vi "Q8381 QRY REF LEVEL.vi"(0 "VISA resource name":refnum<visa-resource-name>, 1 "GPIB Address":u16=8 max=31 step=1) -> (2 "GPIB Status":bool, 3 "REF level data":string, 4 "REF level value":ext format="%.1e")   [LabVIEW 2017]
panel:
  out "program code":string
  # "Query REF LEVEL"
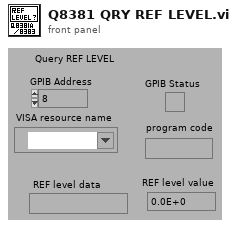
[diagram p1: front panel]
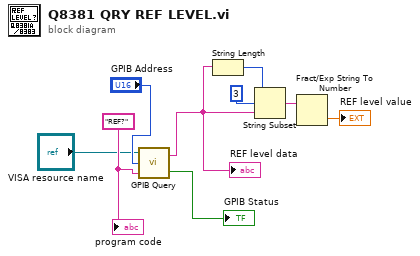
[diagram p0: block diagram]
diagram:
  w2 = "REF?"
  n1 = call "GPIB Query.vi"("Command String"=w2, "Address"="GPIB Address", "VISA resource name"="VISA resource name") -> ("Error"=→"GPIB Status":bool, "Query Data"=w5:string)
  "REF level data" <- w5
  n2 = String Length(string=w5) -> (length=w7:i32)
  n3 = String Subset(string=w5, offset (0)=3, length (rest)=w7) -> (substring=w9:string)
  n4 = Fract/Exp String To Number(string=w9) -> (number=→"REF level value":dbl)  [unwired: 3 in, 1 out]
  "program code" <- w2
